vi "ErrorHelper.vi"(1 "Message":string, 2 "Code":i32, 3 "This VI":refnum<vi>) -> (0 "error out":errorcluster)   [LabVIEW 2011, in "Konvolucio MCAN120803.lvlib"]
uses:
  <instrlib>/Konvolucio MCAN120803/Konvolucio MCAN120803.lvlib
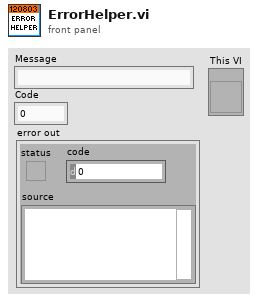
[diagram p1: front panel]
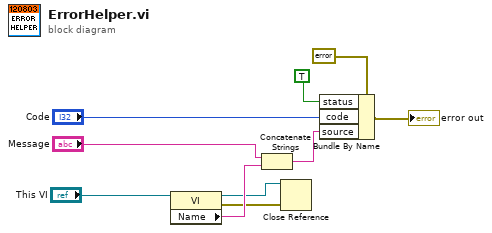
[diagram p0: block diagram]
diagram:
  n1 = property class="VI"(reference="This VI") -> (reference out=w2:refnum<vi>, error out=w1:errorcluster, "Name"=w3:string)  [unwired: 1 in]
  n2 = Concatenate Strings("Message", w3) -> (w9:string)
  n3 = Close Reference(reference=w2, error in (no error)=w1) -> ()  [unwired: 1 out]
  n4 = Bundle By Name(cluster=errorcluster {"status"=FALSE, "code"=0, "source"=""} ("error out"), "status"=TRUE, "code"="Code", "source"=w9) -> (→"error out":errorcluster)
